vi "roboRIO v1.0 Read Encoder.vi"(8 "error in (no error)":errorcluster, 9 "Reset Counter":bool, 10 "Channel":T2, 11 "myRIO Ref In":T3) -> (0 "error out":errorcluster, 1 "Counter Direction":T1, 2 "Counter Value":i32, 3 "myRIO Ref Out":T3, 5 "Overflow?":bool)   [LabVIEW 2021]
uses:
  <vilib>/myRIO/Common/Instrument Driver Framework/Utilities/typedefs/myRIO v1.0 Reference.ctl
  <vilib>/myRIO/Common/Instrument Driver Framework/Utilities/typedefs/Generic FPGA Reference.ctl
  <vilib>/myRIO/Common/Instrument Driver Framework/myRIO v1.0/Encoder/typedefs/Encoder Channels Enum.ctl
  <vilib>/myRIO/Common/Instrument Driver Framework/myRIO v1.0/Encoder/typedefs/Encoder Count Direction Enum.ctl
  <vilib>/myRIO/Common/Instrument Driver Framework/roboRIO v1.0/Encoder/typedefs/roboRIO Encoder Channels FPGA Reference.ctl
  <vilib>/rvi/errors/niLvFpgaAdjustHostInterfaceError.vi
  <vilib>/rvi/interface/nirviReadWriteControl/nirviReadWriteControl.xnode
  <vilib>/rvi/interface/Simulation/niFpgaSimulationCallBeginRW.vi
  NiFpgaLv.dll
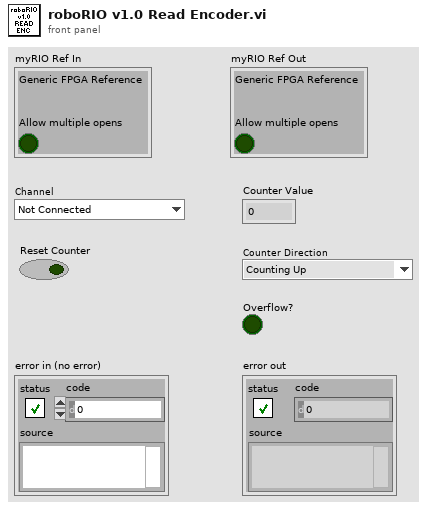
[diagram p1: front panel]
types:
  T1 = typedef "Encoder Count Direction Enum.ctl" = enum16{"Counting Up", "Counting Down"}
  T2 = typedef "Encoder Channels Enum.ctl" = enum16{"Not Connected", "C/ENC0", "C/ENC1", "A/ENC", "A/ENC0", "A/ENC1", "A/ENC2", "A/ENC3", "A/ENC4", "A/ENC5", "A/ENC6", "A/ENC7", "A/ENC8", "A/ENC9", "B/ENC", "B/ENC0", "B/ENC1", "B/ENC2", "B/ENC3", "B/ENC4", "B/ENC5", "B/ENC6", "B/ENC7", "B/ENC8", "B/ENC9", "DIO/ENC0", "DIO/ENC1", "DIO/ENC2", "DIO/ENC3", "DIO/ENC4"}
  T3 = typedef "myRIO v1.0 Reference.ctl" = cluster{"Generic FPGA Reference":T4, "Allow multiple opens":bool}
  T4 = typedef "Generic FPGA Reference.ctl" = refnum<k20>
  T5 = typedef "roboRIO Encoder Channels FPGA Reference.ctl" = refnum<k20>
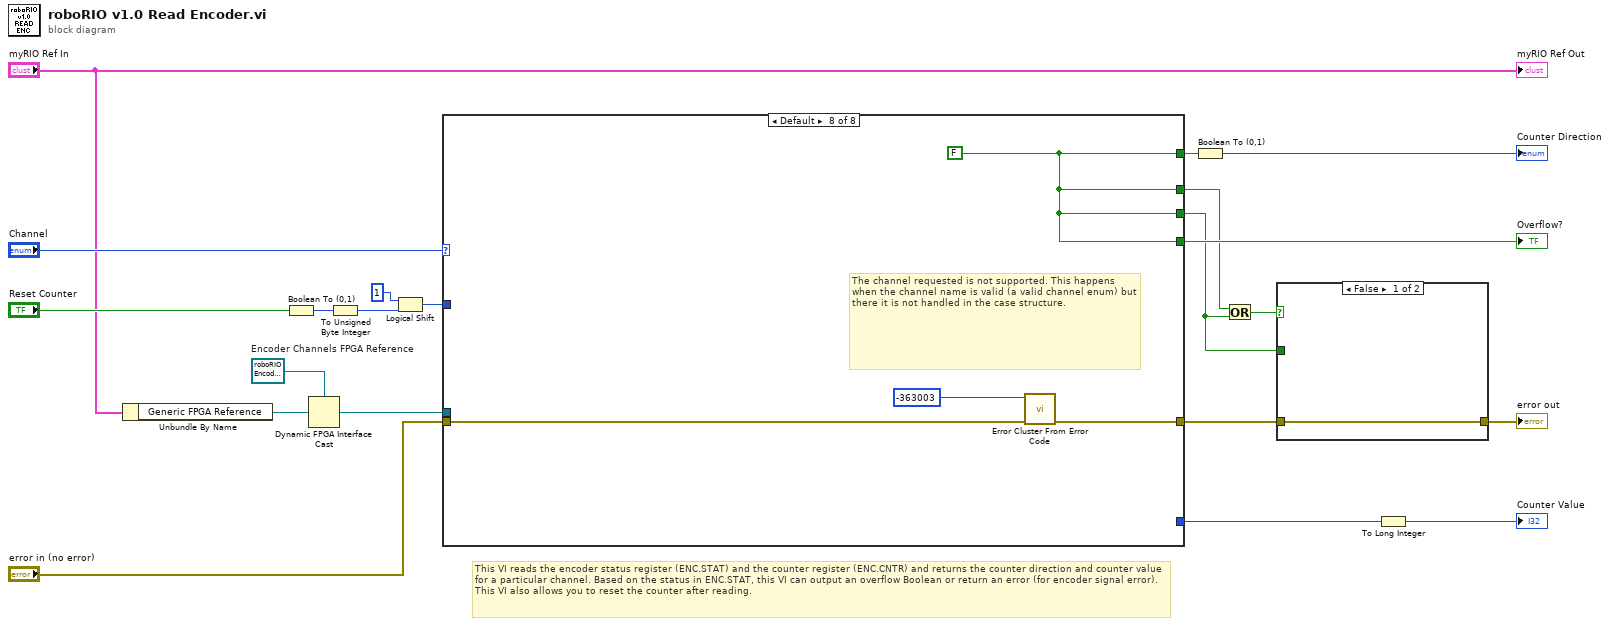
[diagram p0: block diagram]
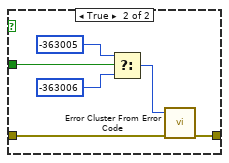
[diagram p2: hidden frame]
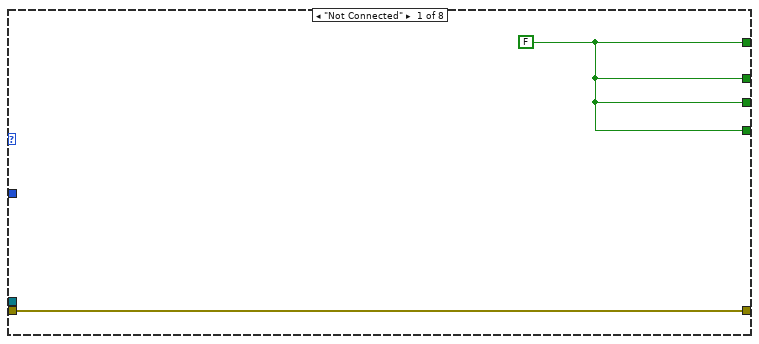
[diagram p3: hidden frame]
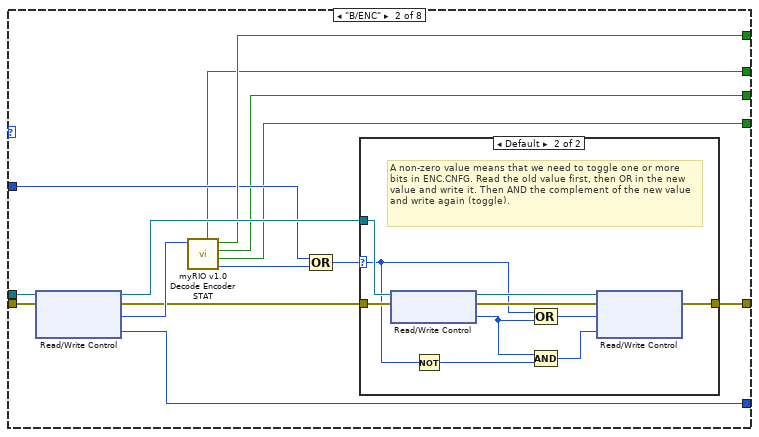
[diagram p4: hidden frame]
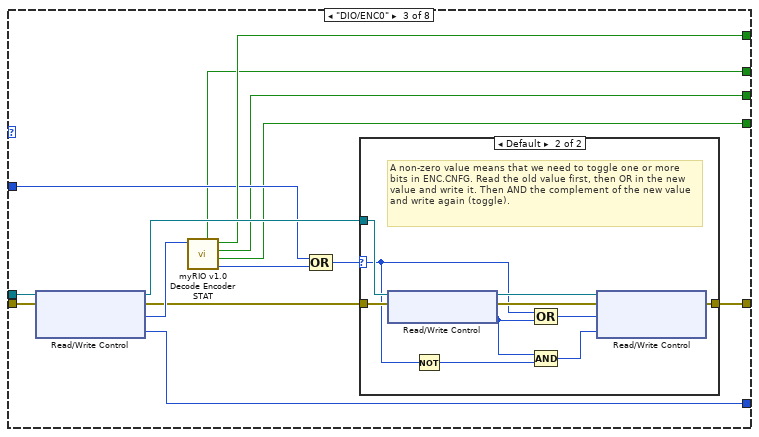
[diagram p6: hidden frame]
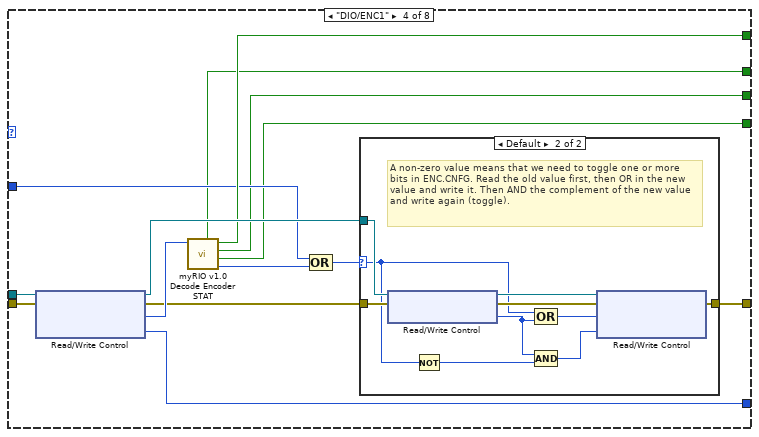
[diagram p8: hidden frame]
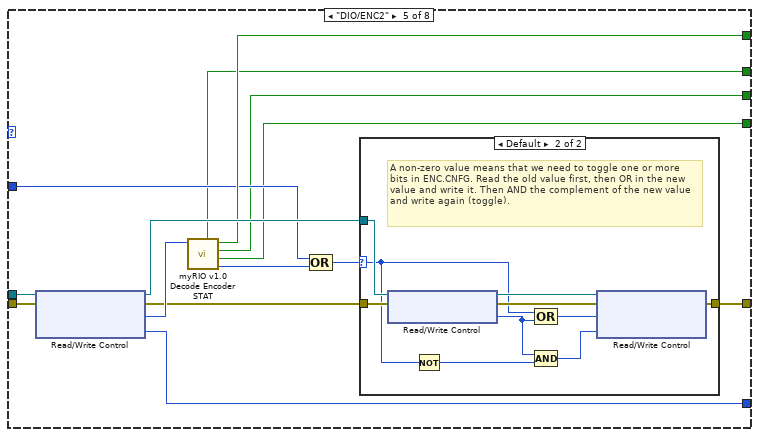
[diagram p10: hidden frame]
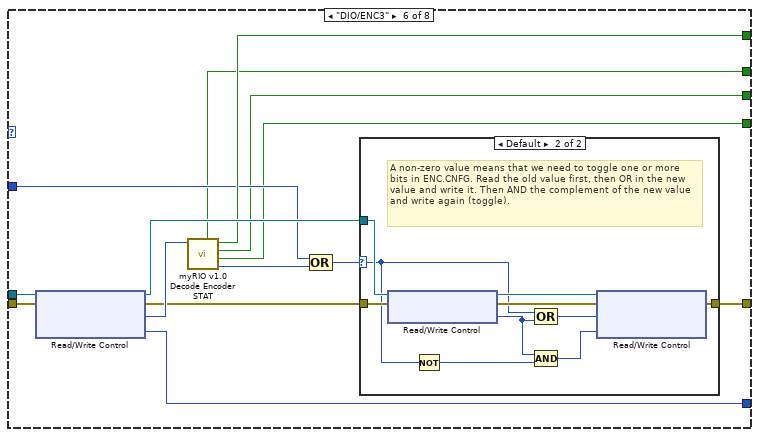
[diagram p12: hidden frame]
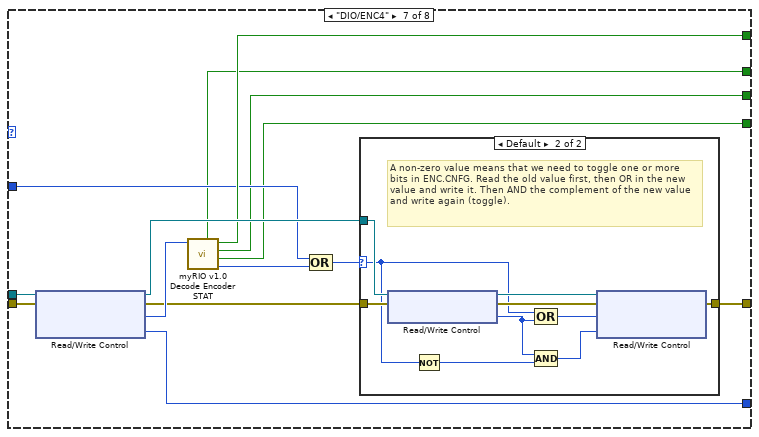
[diagram p14: hidden frame]
diagram:
  w21 = T5 refnum  # Encoder Channels FPGA Reference
  # "This VI reads the encoder status register (ENC.STAT) and the counter register (ENC.CNTR) and returns the counter direction and counter value for a particular channel. Based on the status in ENC.STAT, this VI can output an overflow Boolean or return an error (for encoder signal error). This VI also allows you to reset the counter after reading."
  n1 = Unbundle By Name("myRIO Ref In") -> ("Generic FPGA Reference"=w6:T4)
  n2 = Boolean To (0,1)(Boolean="Reset Counter") -> (0, 1=w7:i16)
  n3 = Dynamic FPGA Interface Cast(Session In=w21, Type=w6) -> (Session Out=w20:T5)
  n4 = To Unsigned Byte Integer(number=w7) -> (unsigned 8bit integer=w8:u8)
  n5 = Logical Shift(y=u8 1, x=w8) -> (x << y=w11:u8)
  n6 = case shown="Default" "Channel" {
    tunnel: "error in (no error)" -> [w23 w36 w61 w86 w111 w136 w161 w175]
    tunnel: [w23 w33 w58 w83 w108 w133 w158 w176] -> w16
    tunnel: w20 -> [_ w37 w62 w87 w112 w137 w162 _]
    tunnel: [w22 w28 w53 w78 w103 w128 w153 w174] -> w13
    tunnel: [_ w32 w57 w82 w107 w132 w157 _] -> w17
    tunnel: w11 -> [_ w27 w52 w77 w102 w127 w152 _]
    tunnel: [w22 w26 w51 w76 w101 w126 w151 w174] -> w1
    tunnel: [w22 w25 w50 w75 w100 w125 w150 w174] -> w9
    tunnel: [w22 w24 w49 w74 w99 w124 w149 w174] -> w3
    frame "Not Connected" {
      w22 = FALSE ("Counting down?")
    }
    frame "B/ENC" {
      n7 = xnode "Read/Write Control"("FPGA VI Reference In"=w37, "error in"=w36) -> ("FPGA VI Reference Out"=w34:T5, "error out"=w29:errorcluster, "ENC.B.STAT"=w35:u8, "ENC.B.CNTR"=w32:u32)
      n8 = call <vilib>:"myRIO v1.0 Decode Encoder STAT.vi"("ENC.STAT"=w35) -> ("ENC.CNFG to write"=w30:u8, "Signed Overflow?"=w25:bool, "Error?"=w26:bool, "Counting down?"=w28:bool, "Signed Overflow Error?"=w24:bool)  [unwired: 6 in]
      n9 = Compound Arithmetic op=OR(w27, w30) -> (w31:u8)
      n10 = case shown="Default" w31 {
        selector: w31 -> [_ w39]
        tunnel: w34 -> [_ w45]
        tunnel: w29 -> [w38 w44]
        tunnel: [w38 w43] -> w33
        frame 0 {
        }
        frame Default {
          # "A non-zero value means that we need to toggle one or more bits in ENC.CNFG. Read the old value first, then OR in the new value and write it. Then AND the complement of the new value and write again (toggle)."
          n11 = xnode "Read/Write Control"("FPGA VI Reference In"=w45, "error in"=w44) -> ("FPGA VI Reference Out"=w47:T5, "error out"=w48:errorcluster, "ENC.B.CNFG"=w41:u8)
          n12 = Not(x=w39) -> (.not. x?=w40:u8)
          n13 = Compound Arithmetic op=OR(w39, w41) -> (w46:u8)
          n14 = Compound Arithmetic op=AND(w41, w40) -> (w42:u8)
          n15 = xnode "Read/Write Control"("FPGA VI Reference In"=w47, "error in"=w48, "ENC.B.CNFG"=w46, "ENC.B.CNFG"=w42) -> ("error out"=w43:errorcluster)  [unwired: 1 out]
        }
      }
    }
    frame "DIO/ENC0" {
      n16 = xnode "Read/Write Control"("FPGA VI Reference In"=w62, "error in"=w61) -> ("FPGA VI Reference Out"=w59:T5, "error out"=w54:errorcluster, "ENC.DIO_0.STAT"=w60:u8, "ENC.DIO_0.CNTR"=w57:u32)
      n17 = call <vilib>:"myRIO v1.0 Decode Encoder STAT.vi"("ENC.STAT"=w60) -> ("ENC.CNFG to write"=w55:u8, "Signed Overflow?"=w50:bool, "Error?"=w51:bool, "Counting down?"=w53:bool, "Signed Overflow Error?"=w49:bool)  [unwired: 6 in]
      n18 = Compound Arithmetic op=OR(w52, w55) -> (w56:u8)
      n19 = case shown="Default" w56 {
        selector: w56 -> [_ w64]
        tunnel: w59 -> [_ w70]
        tunnel: w54 -> [w63 w69]
        tunnel: [w63 w68] -> w58
        frame 0 {
        }
        frame Default {
          # "A non-zero value means that we need to toggle one or more bits in ENC.CNFG. Read the old value first, then OR in the new value and write it. Then AND the complement of the new value and write again (toggle)."
          n20 = xnode "Read/Write Control"("FPGA VI Reference In"=w70, "error in"=w69) -> ("FPGA VI Reference Out"=w72:T5, "error out"=w73:errorcluster, "ENC.DIO_0.CNFG"=w66:u8)
          n21 = Not(x=w64) -> (.not. x?=w65:u8)
          n22 = Compound Arithmetic op=OR(w64, w66) -> (w71:u8)
          n23 = Compound Arithmetic op=AND(w66, w65) -> (w67:u8)
          n24 = xnode "Read/Write Control"("FPGA VI Reference In"=w72, "error in"=w73, "ENC.DIO_0.CNFG"=w71, "ENC.DIO_0.CNFG"=w67) -> ("error out"=w68:errorcluster)  [unwired: 1 out]
        }
      }
    }
    frame "DIO/ENC1" {
      n25 = xnode "Read/Write Control"("FPGA VI Reference In"=w87, "error in"=w86) -> ("FPGA VI Reference Out"=w84:T5, "error out"=w79:errorcluster, "ENC.DIO_1.STAT"=w85:u8, "ENC.DIO_1.CNTR"=w82:u32)
      n26 = call <vilib>:"myRIO v1.0 Decode Encoder STAT.vi"("ENC.STAT"=w85) -> ("ENC.CNFG to write"=w80:u8, "Signed Overflow?"=w75:bool, "Error?"=w76:bool, "Counting down?"=w78:bool, "Signed Overflow Error?"=w74:bool)  [unwired: 6 in]
      n27 = Compound Arithmetic op=OR(w77, w80) -> (w81:u8)
      n28 = case shown="Default" w81 {
        selector: w81 -> [_ w89]
        tunnel: w84 -> [_ w95]
        tunnel: w79 -> [w88 w94]
        tunnel: [w88 w93] -> w83
        frame 0 {
        }
        frame Default {
          # "A non-zero value means that we need to toggle one or more bits in ENC.CNFG. Read the old value first, then OR in the new value and write it. Then AND the complement of the new value and write again (toggle)."
          n29 = xnode "Read/Write Control"("FPGA VI Reference In"=w95, "error in"=w94) -> ("FPGA VI Reference Out"=w97:T5, "error out"=w98:errorcluster, "ENC.DIO_1.CNFG"=w91:u8)
          n30 = Not(x=w89) -> (.not. x?=w90:u8)
          n31 = Compound Arithmetic op=OR(w89, w91) -> (w96:u8)
          n32 = Compound Arithmetic op=AND(w91, w90) -> (w92:u8)
          n33 = xnode "Read/Write Control"("FPGA VI Reference In"=w97, "error in"=w98, "ENC.DIO_1.CNFG"=w96, "ENC.DIO_1.CNFG"=w92) -> ("error out"=w93:errorcluster)  [unwired: 1 out]
        }
      }
    }
    frame "DIO/ENC2" {
      n34 = xnode "Read/Write Control"("FPGA VI Reference In"=w112, "error in"=w111) -> ("FPGA VI Reference Out"=w109:T5, "error out"=w104:errorcluster, "ENC.DIO_2.STAT"=w110:u8, "ENC.DIO_2.CNTR"=w107:u32)
      n35 = call <vilib>:"myRIO v1.0 Decode Encoder STAT.vi"("ENC.STAT"=w110) -> ("ENC.CNFG to write"=w105:u8, "Signed Overflow?"=w100:bool, "Error?"=w101:bool, "Counting down?"=w103:bool, "Signed Overflow Error?"=w99:bool)  [unwired: 6 in]
      n36 = Compound Arithmetic op=OR(w102, w105) -> (w106:u8)
      n37 = case shown="Default" w106 {
        selector: w106 -> [_ w114]
        tunnel: w109 -> [_ w120]
        tunnel: w104 -> [w113 w119]
        tunnel: [w113 w118] -> w108
        frame 0 {
        }
        frame Default {
          # "A non-zero value means that we need to toggle one or more bits in ENC.CNFG. Read the old value first, then OR in the new value and write it. Then AND the complement of the new value and write again (toggle)."
          n38 = xnode "Read/Write Control"("FPGA VI Reference In"=w120, "error in"=w119) -> ("FPGA VI Reference Out"=w122:T5, "error out"=w123:errorcluster, "ENC.DIO_2.CNFG"=w116:u8)
          n39 = Not(x=w114) -> (.not. x?=w115:u8)
          n40 = Compound Arithmetic op=OR(w114, w116) -> (w121:u8)
          n41 = Compound Arithmetic op=AND(w116, w115) -> (w117:u8)
          n42 = xnode "Read/Write Control"("FPGA VI Reference In"=w122, "error in"=w123, "ENC.DIO_2.CNFG"=w121, "ENC.DIO_2.CNFG"=w117) -> ("error out"=w118:errorcluster)  [unwired: 1 out]
        }
      }
    }
    frame "DIO/ENC3" {
      n43 = xnode "Read/Write Control"("FPGA VI Reference In"=w137, "error in"=w136) -> ("FPGA VI Reference Out"=w134:T5, "error out"=w129:errorcluster, "ENC.DIO_3.STAT"=w135:u8, "ENC.DIO_3.CNTR"=w132:u32)
      n44 = call <vilib>:"myRIO v1.0 Decode Encoder STAT.vi"("ENC.STAT"=w135) -> ("ENC.CNFG to write"=w130:u8, "Signed Overflow?"=w125:bool, "Error?"=w126:bool, "Counting down?"=w128:bool, "Signed Overflow Error?"=w124:bool)  [unwired: 6 in]
      n45 = Compound Arithmetic op=OR(w127, w130) -> (w131:u8)
      n46 = case shown="Default" w131 {
        selector: w131 -> [_ w139]
        tunnel: w134 -> [_ w145]
        tunnel: w129 -> [w138 w144]
        tunnel: [w138 w143] -> w133
        frame 0 {
        }
        frame Default {
          # "A non-zero value means that we need to toggle one or more bits in ENC.CNFG. Read the old value first, then OR in the new value and write it. Then AND the complement of the new value and write again (toggle)."
          n47 = xnode "Read/Write Control"("FPGA VI Reference In"=w145, "error in"=w144) -> ("FPGA VI Reference Out"=w147:T5, "error out"=w148:errorcluster, "ENC.DIO_3.CNFG"=w141:u8)
          n48 = Not(x=w139) -> (.not. x?=w140:u8)
          n49 = Compound Arithmetic op=OR(w139, w141) -> (w146:u8)
          n50 = Compound Arithmetic op=AND(w141, w140) -> (w142:u8)
          n51 = xnode "Read/Write Control"("FPGA VI Reference In"=w147, "error in"=w148, "ENC.DIO_3.CNFG"=w146, "ENC.DIO_3.CNFG"=w142) -> ("error out"=w143:errorcluster)  [unwired: 1 out]
        }
      }
    }
    frame "DIO/ENC4" {
      n52 = xnode "Read/Write Control"("FPGA VI Reference In"=w162, "error in"=w161) -> ("FPGA VI Reference Out"=w159:T5, "error out"=w154:errorcluster, "ENC.DIO_4.STAT"=w160:u8, "ENC.DIO_4.CNTR"=w157:u32)
      n53 = call <vilib>:"myRIO v1.0 Decode Encoder STAT.vi"("ENC.STAT"=w160) -> ("ENC.CNFG to write"=w155:u8, "Signed Overflow?"=w150:bool, "Error?"=w151:bool, "Counting down?"=w153:bool, "Signed Overflow Error?"=w149:bool)  [unwired: 6 in]
      n54 = Compound Arithmetic op=OR(w152, w155) -> (w156:u8)
      n55 = case shown="Default" w156 {
        selector: w156 -> [_ w164]
        tunnel: w159 -> [_ w170]
        tunnel: w154 -> [w163 w169]
        tunnel: [w163 w168] -> w158
        frame 0 {
        }
        frame Default {
          # "A non-zero value means that we need to toggle one or more bits in ENC.CNFG. Read the old value first, then OR in the new value and write it. Then AND the complement of the new value and write again (toggle)."
          n56 = xnode "Read/Write Control"("FPGA VI Reference In"=w170, "error in"=w169) -> ("FPGA VI Reference Out"=w172:T5, "error out"=w173:errorcluster, "ENC.DIO_4.CNFG"=w166:u8)
          n57 = Not(x=w164) -> (.not. x?=w165:u8)
          n58 = Compound Arithmetic op=OR(w164, w166) -> (w171:u8)
          n59 = Compound Arithmetic op=AND(w166, w165) -> (w167:u8)
          n60 = xnode "Read/Write Control"("FPGA VI Reference In"=w172, "error in"=w173, "ENC.DIO_4.CNFG"=w171, "ENC.DIO_4.CNFG"=w167) -> ("error out"=w168:errorcluster)  [unwired: 1 out]
        }
      }
    }
    frame Default {
      w174 = FALSE ("Counting down?")
      # "The channel requested is not supported. This happens when the channel name is valid (a valid channel enum) but there it is not handled in the case structure."
      n61 = call <vilib>:"Error Cluster From Error Code.vi"("error in (no error)"=w175, "error code (0)"=-363003) -> ("error out"=w176:errorcluster)  [unwired: 7 in]
    }
  }
  "Overflow?" <- w9
  n62 = Boolean To (0,1)(Boolean=w13) -> (0, 1=→"Counter Direction":i16)
  n63 = Or(x=w3, y=w1) -> (x .or. y?=w2:bool)
  n64 = case shown="False" w2 {
    tunnel: w16 -> [w178 w183]
    tunnel: [w178 w184] -> w15
    tunnel: w1 -> [_ w182]
    frame False {
    }
    frame True {
      n65 = Select(t=-363005 ("error code (0)"), s=w182, f=-363006 ("error code (0)")) -> (s? t:f=w180:i32)
      n66 = call <vilib>:"Error Cluster From Error Code.vi"("error in (no error)"=w183, "error code (0)"=w180) -> ("error out"=w184:errorcluster)  [unwired: 7 in]
    }
  }
  "error out" <- w15
  n67 = To Long Integer(number=w17) -> (32bit integer=→"Counter Value":i32)
  "myRIO Ref Out" <- "myRIO Ref In"
